vi "Sample  test.vi"() -> ()   [LabVIEW 2022 SP3]
panel:
  out "x+y":dbl
  in  "Numeric 2":dbl
  in  "Numeric":dbl
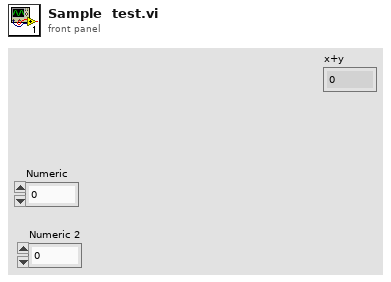
[diagram p1: front panel]
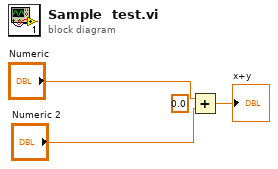
[diagram p0: block diagram]
diagram:
  (unwired) 0.0 ("x+y")
  n1 = Add(x="Numeric", y="Numeric 2") -> (x+y=→"x+y":dbl)
